vi "Conversion.vi"(11 "Sorting Threshold":dbl) -> (2 "Numeric":dbl, 3 "Numeric 2":i16)   [LabVIEW 2017]
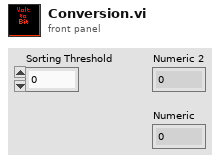
[diagram p1: front panel]
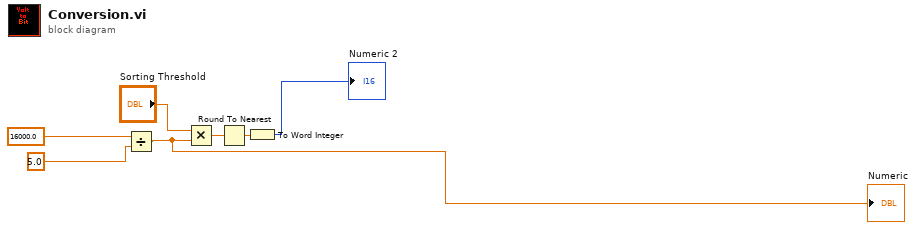
[diagram p0: block diagram]
diagram:
  n1 = Divide(x=16000.0, y=5.0) -> (x/y=w6:dbl)
  "Numeric" <- w6
  n2 = Multiply(x="Sorting Threshold", y=w6) -> (x*y=w2:dbl)
  n3 = Round To Nearest(number=w2) -> (nearest integer value=w3:dbl)
  n4 = To Word Integer(number=w3) -> (16bit integer=→"Numeric 2":i16)
